vi "WORD.ReportGenerator.Chapter.vi"(8 "error in (no error)":errorcluster, 9 "Font":T1, 10 "Chapter":string, 11 "NI_report in":refnum<class "NI_report.lvclass">) -> (0 "error out":errorcluster, 3 "NI_report out":refnum<class "NI_report.lvclass">)   [LabVIEW 2019, in "Tools.lvlib"]
uses:
  <vilib>/Utility/NIReport.llb/NI_report.lvclass
  <vilib>/Utility/NIReport.llb/Append Report Text (str wrap).vi
  Tools.lvlib
  <vilib>/addons/_office/NI_ReportGenerationToolkit.lvlib
  <vilib>/Utility/NIReport.llb/Word/NI_Word.lvclass
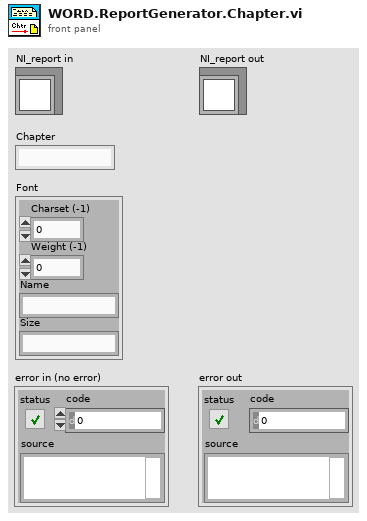
[diagram p1: front panel]
types:
  T1 = cluster{"Charset (-1)":i16, "Weight (-1)":i16, "Name":string, "Size":string}
  T2 = cluster{"Italic":enum16{"Italic Unchanged", "Italic On", "Italic Off"}, "Strike Through":enum16{"Strike Through Unchanged", "Strike Through On", "Strike Through Off"}, "Underline":enum16{"Underline Unchanged", "Underline On", "Underline Off"}, "Bold":enum16{"Bold Unchanged", "Bold On", "Bold Off"}}
  T3 = cluster{"Alignment":enum16{"Left", "Centered", "Right", "Justify"}, "Left":dbl, "Right":dbl, "Special":enum16{"(none)", "First line", "Hanging"}, "By":dbl, "Before":dbl, "After":dbl, "Line spacing":enum16{"Single", "1,5 lines", "Double", "At least", "Exactly", "Multiple"}, "At":dbl}
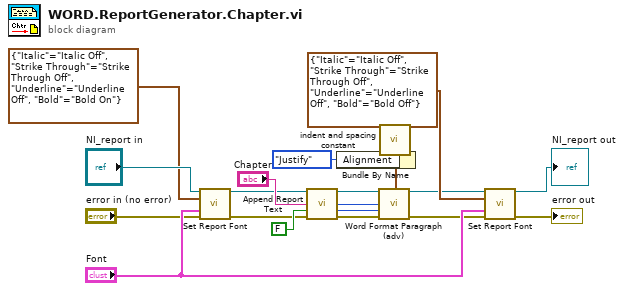
[diagram p0: block diagram]
diagram:
  n1 = call-dynamic "Set Report Font.vi"("report in"="NI_report in", "text options"=T2 {"Italic"=enum."Italic Off", "Strike Through"=enum."Strike Through Off", "Underline"=enum."Underline Off", "Bold"=enum."Bold On"}, "font settings"="Font", "error in (no error)"="error in (no error)") -> ("report out"=w11:refnum<class "NI_report.lvclass">, "error out"=w12:errorcluster)  [unwired: 9 in, 1 out]
  n2 = call-poly <vilib>:"Append Report Text.vi"("report in"=w11, "text"="Chapter", "append on new line? (F)"=FALSE, "error in (no error)"=w12) -> ("report out"=w7:refnum<class "NI_report.lvclass">, "start out (Word)"=w5:i32, "end out (Word)"=w4:i32, "error out"=w3:errorcluster)  [unwired: 8 in]
  n3 = call <vilib>:"indent and spacing constant.vi"() -> ("indent and spacing"=w8:T3)
  n4 = Bundle By Name(cluster=w8, "Alignment"=enum16{"Left", "Centered", "Right", "Justify"}."Justify") -> (w9:T3)
  n5 = call <vilib>:"Word Format Paragraph (adv).vi"("report in"=w7, "indent and spacing"=w9, "start (-1)"=w5, "end (-1)"=w4, "error in (no error)"=w3) -> ("report out"=w6:refnum<class "NI_report.lvclass">, "error out"=w2:errorcluster)  [unwired: 2 in, 7 out]
  n6 = call-dynamic "Set Report Font.vi"("report in"=w6, "text options"=T2 {"Italic"=enum."Italic Off", "Strike Through"=enum."Strike Through Off", "Underline"=enum."Underline Off", "Bold"=enum."Bold Off"}, "font settings"="Font", "error in (no error)"=w2) -> ("report out"=→"NI_report out":refnum<class "NI_report.lvclass">, "error out"=→"error out":errorcluster)  [unwired: 9 in, 1 out]
